vi "getRegisters.vi"(0 "AddressSpace in":refnum<class "AddressSpace.lvclass">) -> (4 "CntlRegisters":T1={"Parameters"="Parameters", "VDCLinkToP_PISettings"="Range", "ID_to_VD_PISettings"="gains", "IQ_to_VQ_PISettings"="Setpoints", "VDCLink"="VDCLink", "P"="VDCLink", "Q"="VDCLink", "pf"="VDCLink"})   [LabVIEW 2017, in "ActiveFrontEnd.lvlib" / "AddressSpace.lvclass"]
uses:
  AddressSpace.lvclass
  ControllerRegisters.ctl
  AddressSpace.lvclass/AddressSpace.ctl
  ActiveFrontEnd.lvlib
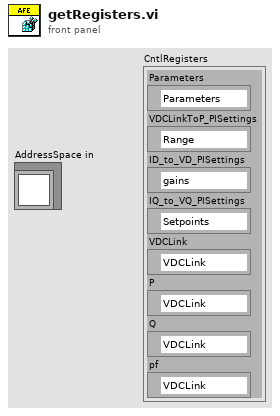
[diagram p1: front panel]
types:
  T1 = typedef "ActiveFrontEnd.lvlib/ControllerRegisters.ctl" = cluster{"Parameters":refnum<k21>, "VDCLinkToP_PISettings":refnum<k21>, "ID_to_VD_PISettings":refnum<k21>, "IQ_to_VQ_PISettings":refnum<k21>, "VDCLink":refnum<k21>, "P":refnum<k21>, "Q":refnum<k21>, "pf":refnum<k21>}
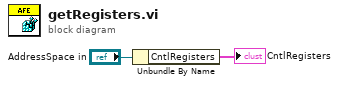
[diagram p0: block diagram]
diagram:
  n1 = Unbundle By Name("AddressSpace in") -> ("CntlRegisters"=→"CntlRegisters":T1)
